vi "Do.vi"(8 "error in (no error)":errorcluster, 10 "Actor in":refnum<class "Actor.lvclass">, 11 "ShutdownTimedOut Msg":refnum<class "ShutdownTimedOut Msg.lvclass">) -> (0 "error out":errorcluster, 2 "Actor out":refnum<class "Actor.lvclass">)   [LabVIEW 2020, in "MGI-Panel Actor.lvlib" / "AdvancedActor.lvlib" / "ShutdownTimedOut Msg.lvclass"]
doc: "This VI delivers the message to the actor by calling the appropriate method(s) on the actor."
uses:
  ShutdownTimedOut Msg.lvclass
  <vilib>/ActorFramework/Actor/Actor.lvclass
  <vilib>/Utility/error.llb/Error Cluster From Error Code.vi
  <vilib>/ErrorRing/Error Ring.xnode
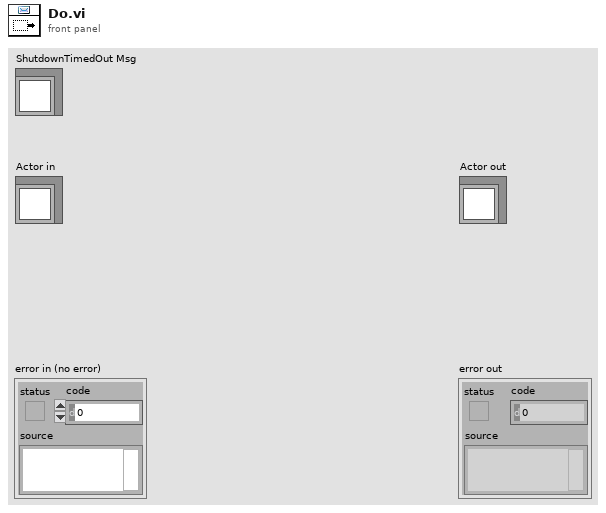
[diagram p1: front panel]
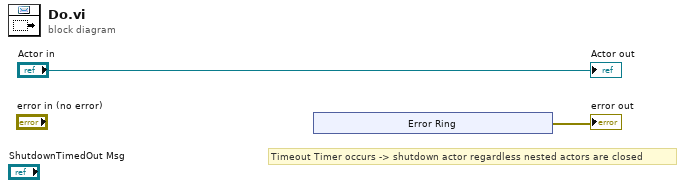
[diagram p0: block diagram]
diagram:
  # "Timeout Timer occurs -> shutdown actor regardless nested actors are closed"
  n1 = xnode "Error Ring"() -> ("error out"=→"error out":errorcluster)
  "Actor out" <- "Actor in"
